vi "GetAbsorptionCrossSectionsFromLinearLineRegression.vi"(3 "Extinction ExtinctionUncertainity Size parameter and Number ofS sizes 2":T1={"PAS amplitude"=[], "PAS amp Uncertainty"=[], "Size parameters"=[], "Number ofSizes"=0.0, "GeometricCrossSection"=[], "Wave Length"=0.0, "SMPS Sizes"=[], "Concentration"=[], "Double Charge Correction"=FALSE, "Extincation Factor"=1.0, "Diameter Factor"=1.0, "Diameter Offset"=0.0, "Extinction Factor Flag"=FALSE, "Diameter Factor Flag"=FALSE, "Diameter Offset Flag"=FALSE, "Sizes"=[], "ExtinctionOrAbsorptionOrScattering"=0, "Concentration(#/cc)"=[]} {"ExtinctionOrAbsorptionOrScattering" scale=0.0..2.0}, 4 "refractive index, imaginary":dbl=0.037 format="%.5f", 5 "refractive index, real":dbl=1.567 format="%.5f") -> (0 "Predicted Extinction/Absorption Cross Section":dbl[](array[numeric]), 1 "Expected Extinction/Absorption Cross Section Uncer":dbl[](array[numeric]), 2 "Expected Extinction/Absorption Cross Section":dbl[](array[numeric]))   [LabVIEW 2013]
uses:
  BaesDataTypeDefinition.ctl
  <vilib>/Analysis/6fits.llb/Curve Fitting Criteria.ctl
  <vilib>/Analysis/NI_AALPro.lvlib
panel:
  out "Absorption Coef Predicted Mie":dbl[](array[numeric])
  out "Offset":dbl
  out "slope":dbl
  # "Mie scattering demo program, August 2005, by Martin Fierz (martin@fierz.ch)\n\nThis VI demonstrates the usage of mie2.dll; a dynamic-link-library which you can call in your LabView program.\nThe demo lets you select the refractive index of a sphere, and the size parameter and computes total scattering,\ntotal extinction and angular distribution of the scattered light for p-, s- and unpolarized light.\nMie2.dll uses the Bohren-Huffman Mie code."
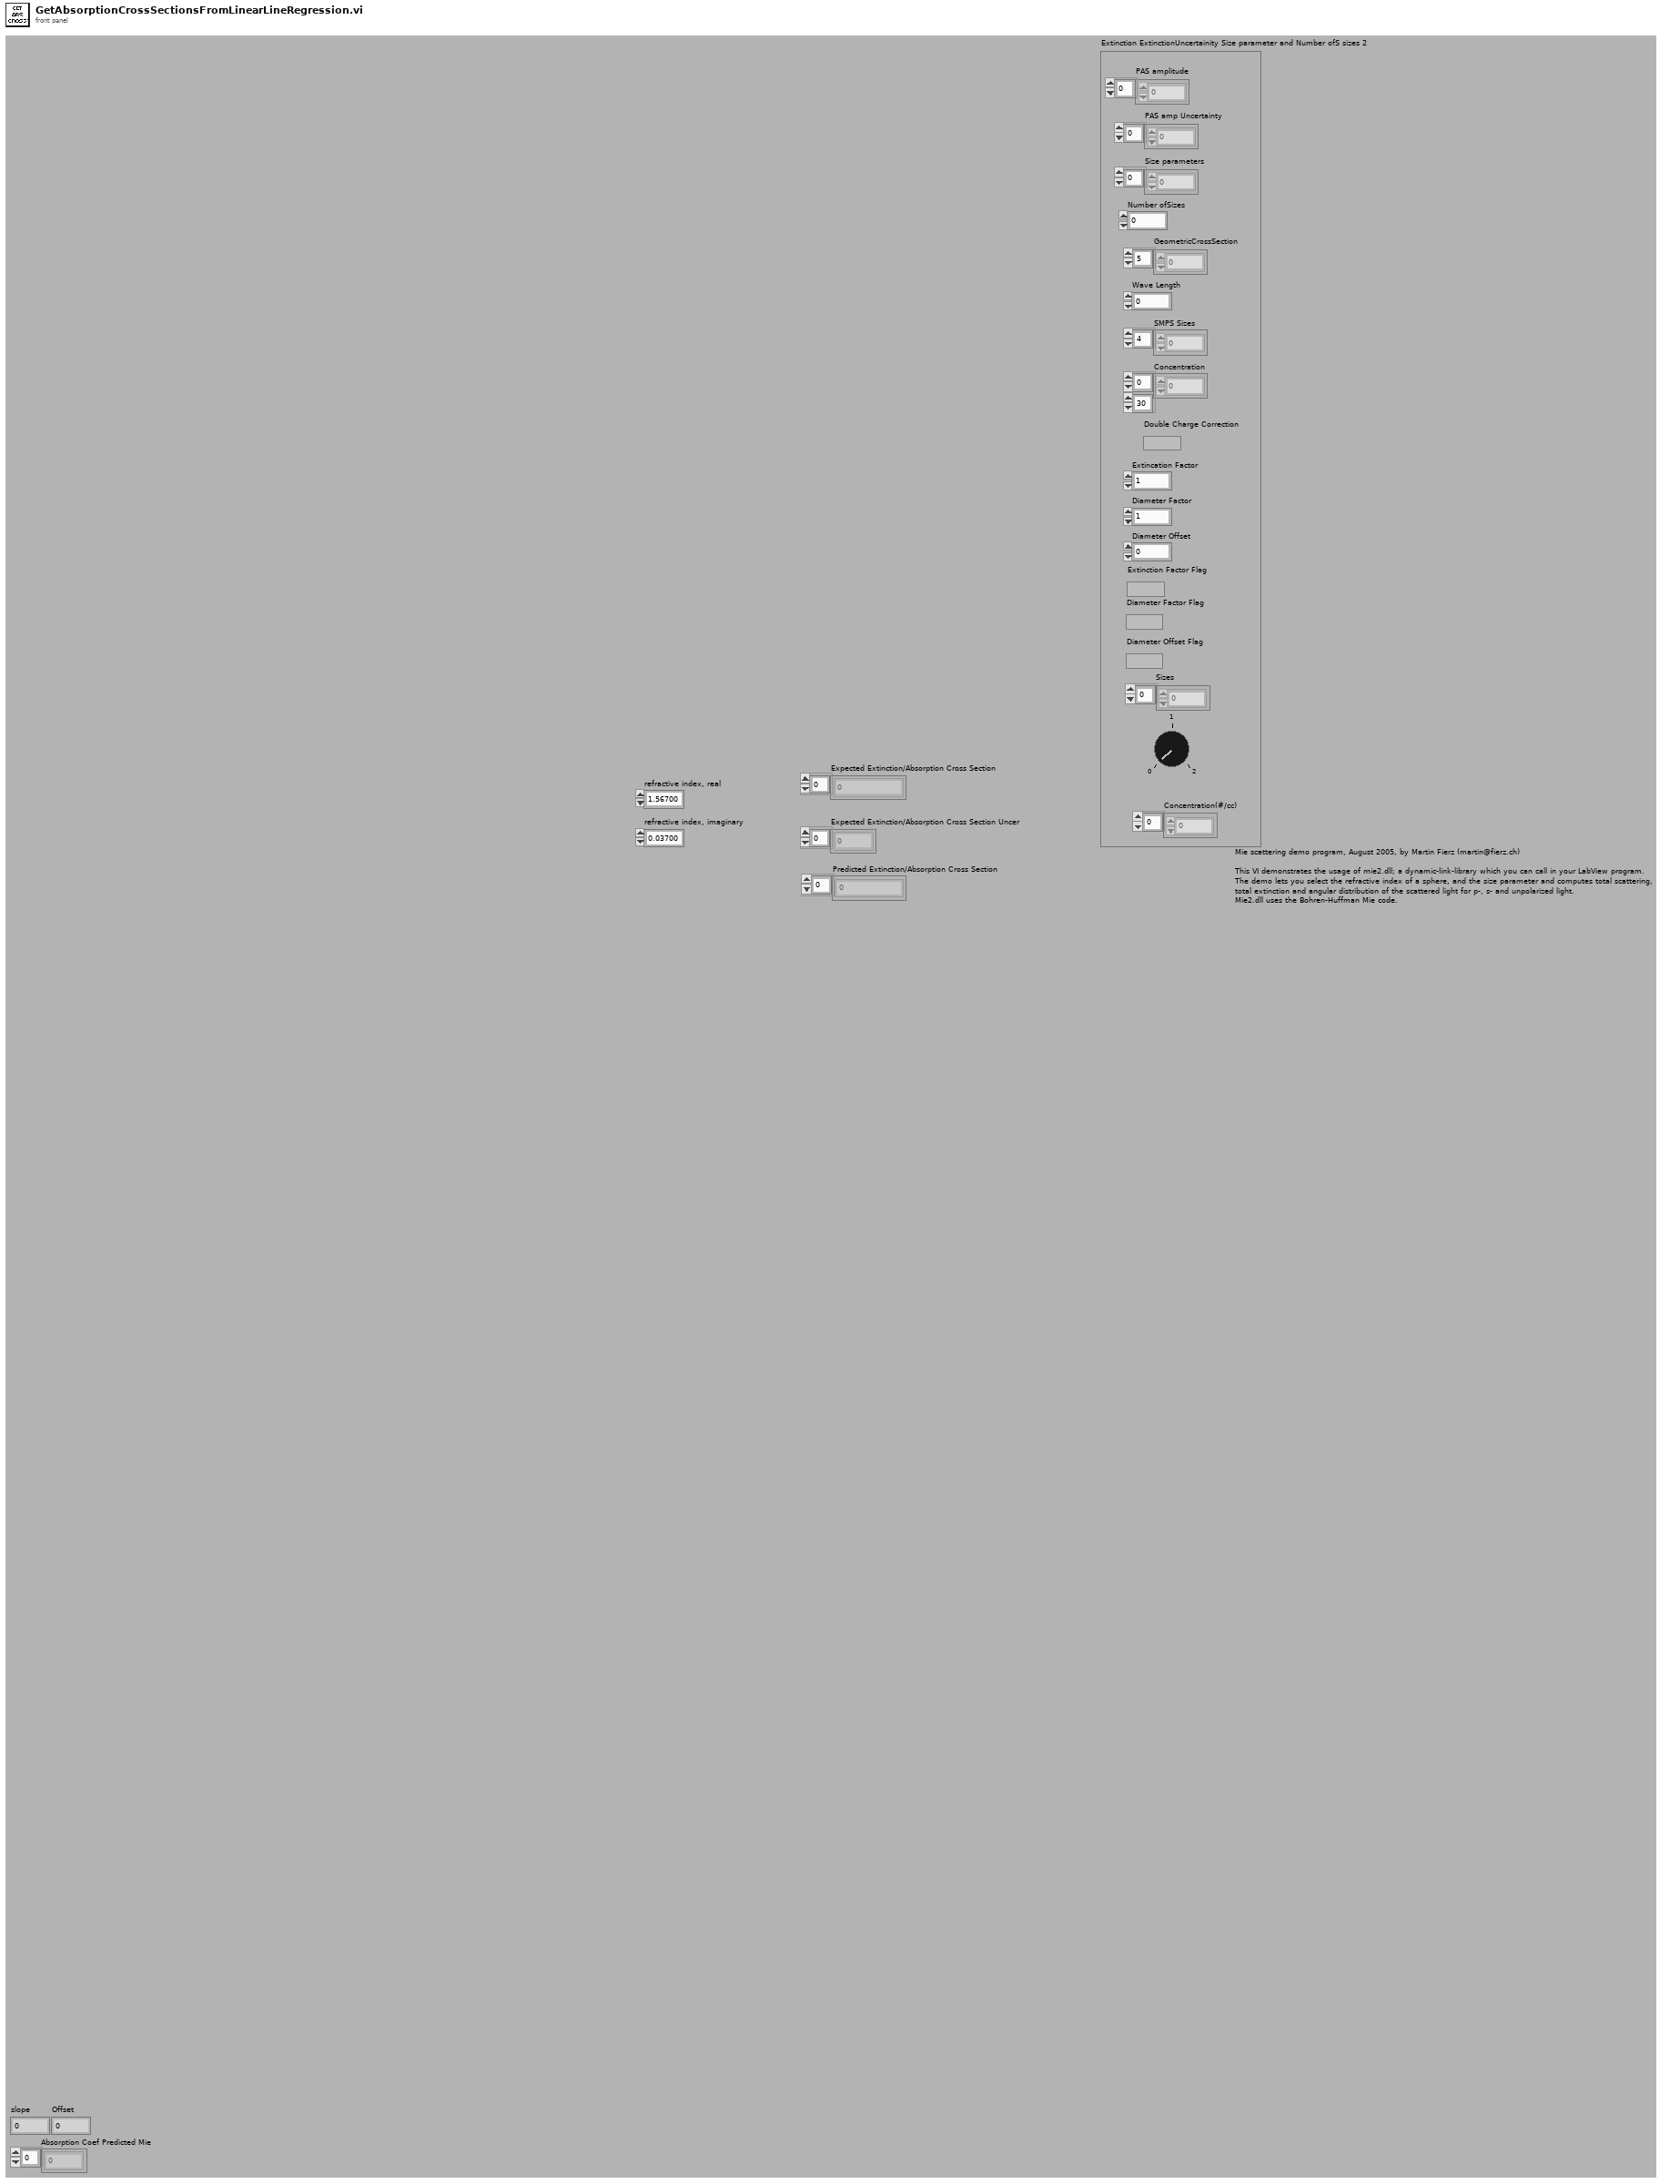
[diagram p1: front panel]
types:
  T1 = typedef "BaesDataTypeDefinition.ctl" = cluster{"PAS amplitude":dbl[], "PAS amp Uncertainty":dbl[], "Size parameters":dbl[], "Number ofSizes":dbl, "GeometricCrossSection":dbl[], "Wave Length":dbl, "SMPS Sizes":dbl[], "Concentration":dbl[][], "Double Charge Correction":bool, "Extincation Factor":dbl, "Diameter Factor":dbl, "Diameter Offset":dbl, "Extinction Factor Flag":bool, "Diameter Factor Flag":bool, "Diameter Offset Flag":bool, "Sizes":dbl[], "ExtinctionOrAbsorptionOrScattering":i8, "Concentration(#/cc)":dbl[]}
  T2 = typedef "NI_AALPro.lvlib/Curve Fitting Criteria.ctl" = u16
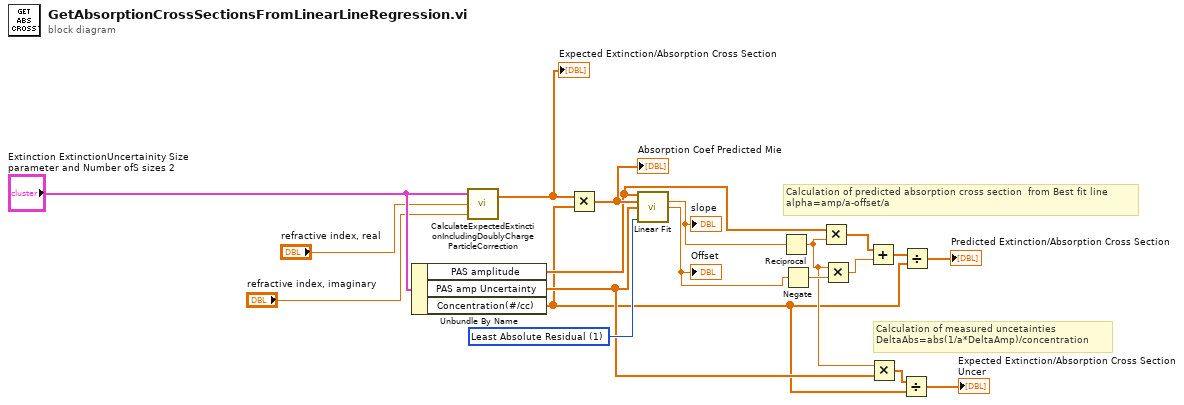
[diagram p0: block diagram]
diagram:
  w16 = T2 1 items=["Least Square", "Least Absolute Residual", "Bisquare"] ("method")
  # "Calculation of measured uncetainties\nDeltaAbs=abs(1/a*DeltaAmp)/concentration"
  # "Calculation of predicted absorption cross section  from Best fit line\nalpha=amp/a-offset/a"
  n1 = Unbundle By Name("Extinction ExtinctionUncertainity Size parameter and Number ofS sizes 2") -> ("PAS amplitude"=w12:dbl[], "PAS amp Uncertainty"=w5:dbl[], "Concentration(#/cc)"=w2:dbl[])
  n2 = call "CalculateExpectedExtinctionIncludingDoublyChargeParticleCorrection.vi"("refractive index, imaginary"="refractive index, imaginary", "refractive index, real"="refractive index, real", "Extinction ExtinctionUncertainity Size parameter and Number ofS sizes"="Extinction ExtinctionUncertainity Size parameter and Number ofS sizes 2") -> ("Expected Extinction/Absorption Cross Section"=w14:sgl[])  [unwired: 1 out]
  "Expected Extinction/Absorption Cross Section" <- w14
  n3 = Multiply(x=w14, y=w2) -> (x*y=w15:dbl[])
  "Absorption Coef Predicted Mie" <- w15
  n4 = call <vilib>:"Linear Fit.vi"("Y"=w12, "X"=w15, "Weight"=w5, "method"=w16) -> ("slope"=w13:dbl, "intercept"=w11:dbl)  [unwired: 7 in, 3 out]
  "slope" <- w13
  "Offset" <- w11
  n5 = Reciprocal(x=w13) -> (1/x=w4:dbl)
  n6 = Negate(x=w11) -> (-x=w10:dbl)
  n7 = Multiply(x=w12, y=w4) -> (x*y=w9:dbl[])
  n8 = Multiply(x=w4, y=w10) -> (x*y=w8:dbl)
  n9 = Add(x=w9, y=w8) -> (x+y=w7:dbl[])
  n10 = Multiply(x=w4, y=w5) -> (x*y=w3:dbl[])
  n11 = Divide(x=w3, y=w2) -> (x/y=→"Expected Extinction/Absorption Cross Section Uncer":dbl[])
  n12 = Divide(x=w7, y=w2) -> (x/y=→"Predicted Extinction/Absorption Cross Section":dbl[])
